vi "c DMC60C Create1.vi"(8 "error in (no error)":errorcluster, 11 "deviceNumber":i32) -> (0 "error out":errorcluster, 3 "function return":i32)   [LabVIEW 2018, in "DMC60C.lvlib"]
doc: "Create a DMC60 Object in memory.\n\n\n\n\n\n\n\n\nint c_DMC60C_Create1(int deviceNumber);"
uses:
  <vilib>/Rock Robotics/WPI/ThirdParty/TopLevel/DMC60C/DMC60C.lvlib
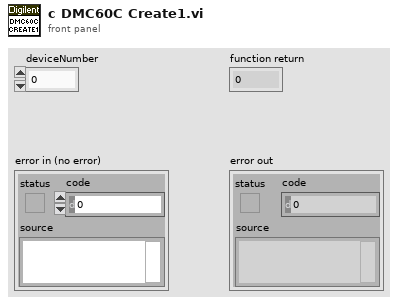
[diagram p1: front panel]
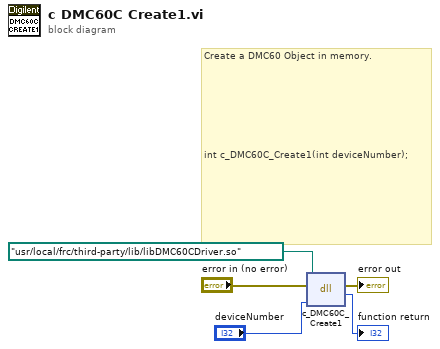
[diagram p0: block diagram]
diagram:
  # "Create a DMC60 Object in memory.\n\n\n\n\n\n\n\n\nint c_DMC60C_Create1(int deviceNumber);"
  n1 = dll-call lib="usr/lib/libdmc60c.so" fn="c_DMC60C_Create1"(path in=path "/usr/local/frc/third-party/lib/libDMC60CDriver.so", error in="error in (no error)", "deviceNumber"="deviceNumber") -> (error out=→"error out":errorcluster, "return type"=→"function return":i32)  [unwired: 2 in, 1 out]
